vi "test-tdms write.vi"() -> ()   [LabVIEW 2014]
uses:
  <vilib>/rvi/interface/nirviOpenFPGA/nirviOpenFPGA.xnode
  FPGA Bitfiles/mySynth_FPGATarget_FPGAMain_WASpsvx+XwM.lvbitx
  FPGA Main.vi
  <vilib>/FPGAPlugInAG/myRIO-1900/niLvFpga_Open_myRIO-1900.vi
  <vilib>/rvi/interface/common/dynamic/niFpgaDynamicAddResources.vi
  <vilib>/rvi/interface/nirviCloseFPGA/nirviCloseFPGA.xnode
  <vilib>/FPGAPlugInAG/Dynamic/niLvFpga_Close_Dynamic.vi
  Controls/Track Enable.ctl
  Controls/Audio In.ctl
panel:
  out "Array":i32[](array[numeric])
  in  "error in":errorcluster
  out "error out":errorcluster
  in  "stop":bool
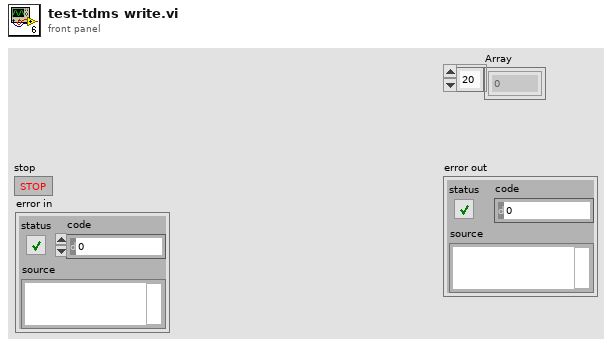
[diagram p1: front panel]
types:
  T1 = typedef "Track (File) References.ctl" = cluster{"Track_1_Ref":refnum<k34>, "Track_2_Ref":refnum<k34>, "Track_3_Ref":refnum<k34>, "Track_4_Ref":refnum<k34>, "Track_Name_1":string, "Track_Name_2":string, "Track_Name_3":string, "Track_Name_4":string}
  T2 = typedef "Audio In.ctl" = cluster{"AudioIn/Left (N Samples)":i16[], "AudioIn/Right (N Samples)":i16[]}
  T3 = typedef "Track Enable.ctl" = cluster{"Track_1 _Enable ":bool, "Track_2 _Enable ":bool, "Track_3 _Enable ":bool, "Track_4 _Enable ":bool}
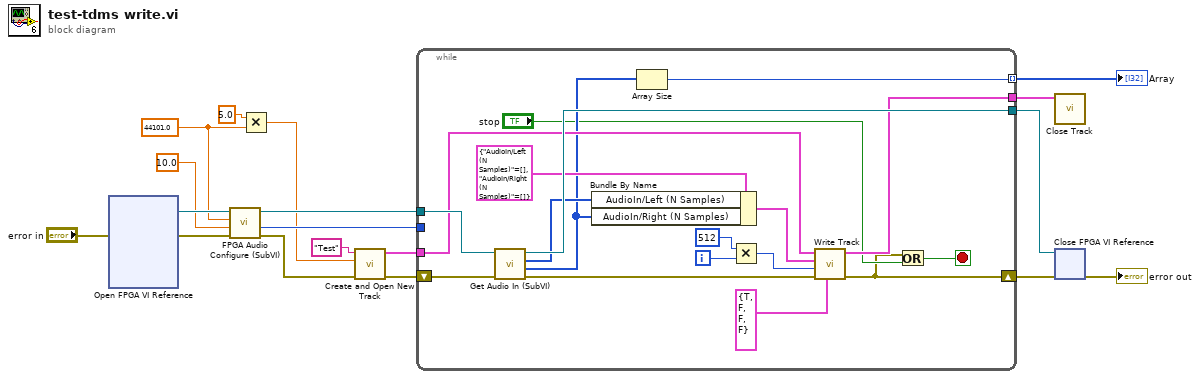
[diagram p0: block diagram]
diagram:
  w11 = 44101.0 ("Audio Sample Rate (Hz)")
  n1 = xnode "Open FPGA VI Reference"("error in"="error in") -> ("FPGA VI Reference Out"=w18:refnum<k20>, "error out"=w13:errorcluster)  [unwired: 1 in]
  n2 = call "FPGA Audio Configure (SubVI).vi"("error in (no error)"=w13, "Read Rate (Hz)"=10.0, "Audio Sample Rate (Hz)"=w11, "Refnum in"=w18) -> ("error out"=w2:errorcluster, "Required loop period (ms)"=w12:u32, "Refnum out"=w9:refnum<k20>)  [unwired: 4 in, 1 out]
  n3 = Multiply(x=5.0, y=w11) -> (x*y=w6:dbl)
  n4 = call "Create and Open New Track.vi"("Error In"=w2, "Samples Per Channel"=w6, "Track Name"="Test") -> ("Error Out"=w1:errorcluster, "Track (File) References"=w7:T1)  [unwired: 7 in]
  n5 = while {
    shift-right: [w20] -> w16
    shift-left: w1 -> [w32]
    tunnel: w12 -> [_]
    tunnel: w9 -> [w34]
    tunnel: w7 -> [w29]
    tunnel: [w33] -> w5
    tunnel: [w23] -> w4 mode=indexing
    tunnel: [w22] -> w3
    i -> [w36]
    stop <- w19 stop-if-true
    n6 = call "Get Audio In (SubVI).vi"("error in (no error)"=w32, "Refnum in"=w34) -> ("error out"=w31:errorcluster, "Right Audio In"=w24:i16[], "Left Audio In"=w27:i16[], "Refnum out"=w33:refnum<k20>)  [unwired: 6 in]
    n7 = Bundle By Name(cluster=T2 {"AudioIn/Left (N Samples)"=[], "AudioIn/Right (N Samples)"=[]} ("Audio In"), "AudioIn/Left (N Samples)"=w27, "AudioIn/Right (N Samples)"=w24) -> (w26:T2)
    n8 = Array Size(array=w24) -> (size(s)=w23:i32)
    n9 = Multiply(x=512, y=w36) -> (x*y=w25:i32)
    n10 = call "Write Track.vi"(6:T3 {"Track_1 _Enable "=TRUE, "Track_2 _Enable "=FALSE, "Track_3 _Enable "=FALSE, "Track_4 _Enable "=FALSE} ("Track Enable"), "Error In"=w31, "Write Position"=w25, "Audio In"=w26, "Track (File) References In"=w29) -> ("Error Out"=w20:errorcluster, "Track (File) References Out"=w22:T1)  [unwired: 5 in]
    n11 = Or(x=w20, y="stop") -> (x .or. y?=w19:bool)
  }
  "Array" <- w4
  n12 = call "Close Track.vi"("Track (File) References"=w3) -> ()  [unwired: 10 in, 1 out]
  n13 = xnode "Close FPGA VI Reference"("FPGA VI Reference In"=w5, "error in"=w16) -> ("error out"=→"error out":errorcluster)
